vi "set Font.vi"(8 "error in (no error)":errorcluster, 9 "Font":cluster{"Font":string, "Size":i32}={"Font"="Consolas", "Size"=8}, 10 "Style index":i32, 11 "ScintillaNET in":refnum<class "ScintillaNET.lvclass">) -> (0 "error out":errorcluster, 3 "ScintillaNET out":refnum<class "ScintillaNET.lvclass">)   [LabVIEW 2018, in "ScintillaNET.lvclass"]
uses:
  ScintillaNET.lvclass
  ScintillaNET.lvclass/ScintillaNET.ctl
  D:/project/hobby/LF2R/LabVIEW/source/ScintillaNET/dll/ScintillaNET.dll
  dll/ScintillaNET.dll
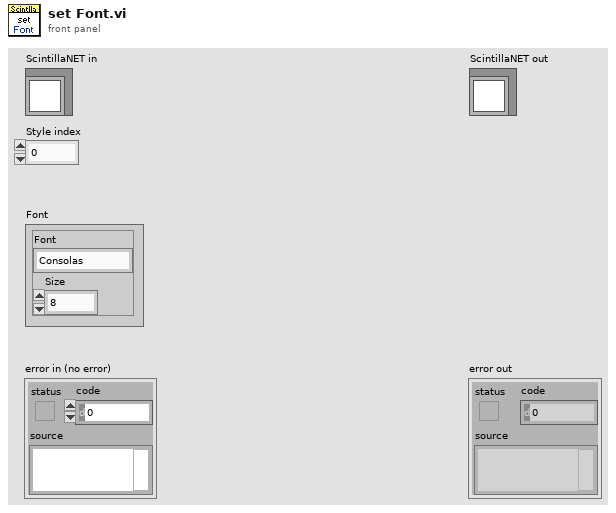
[diagram p1: front panel]
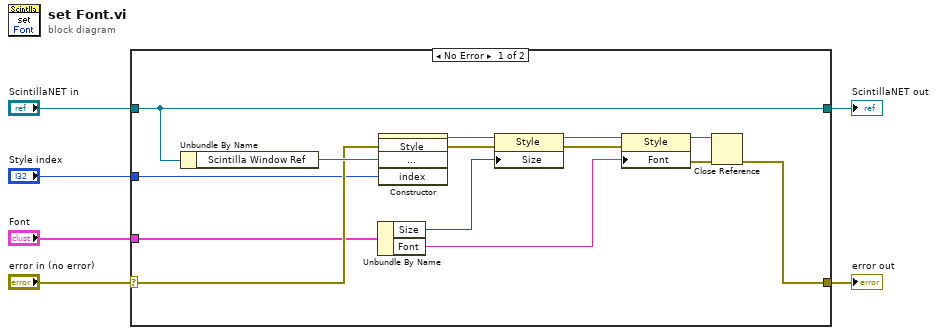
[diagram p0: block diagram]
diagram:
  n1 = case shown="No Error" "error in (no error)" {
    selector: "error in (no error)" -> [w12 w22]
    tunnel: [w7 w22] -> w5
    tunnel: [w13 w21] -> w3
    tunnel: "ScintillaNET in" -> [w13 w21]
    tunnel: "Style index" -> [w11 _]
    tunnel: "Font" -> [w10 _]
    frame No Error {
      n2 = Unbundle By Name(w13) -> ("Scintilla Window Ref"=w14:refnum<k24>)
      n3 = Unbundle By Name(w10) -> ("Size"=w9:i32, "Font"=w8:string)
      n4 = constructor class="Style"(error in=w12, "scintilla"=w14, "index"=w11) -> (reference out=w20:refnum<k24>, error out=w19:errorcluster)  [unwired: 2 in, 3 out]
      n5 = property class="Style"(reference=w20, error in=w19, "Size"=w9) -> (reference out=w18:refnum<k24>, error out=w17:errorcluster)
      n6 = property class="Style"(reference=w18, error in=w17, "Font"=w8) -> (reference out=w16:refnum<k24>, error out=w15:errorcluster)
      n7 = Close Reference(reference=w16, error in (no error)=w15) -> (error out=w7:errorcluster)
    }
    frame Error {
    }
  }
  "error out" <- w5
  "ScintillaNET out" <- w3
